vi "Write Graph Properties.vi"(0 "Config File":path, 7 "WFGraph Refnum":refnum<vi>, 9 "Section":string, 11 "error in (no error)":errorcluster) -> (15 "error out":errorcluster)   [LabVIEW 2020]
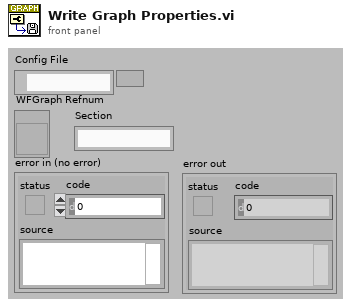
[diagram p1: front panel]
types:
  T1 = typedef "Graph Properties.ctl" = cluster{"X-axis":T2, "Y-axis":T2, "Plot Properties":T3[]}
  T2 = typedef "Axis Properties.ctl" = cluster{"Min":dbl, "Max":dbl, "Fit":u8}
  T3 = typedef "Plot Properties.ctl" = cluster{"Line Style":u8, "Line Width":u8, "Plot Color":u32, "Point Style":u8, "Point color":u32, "Interp":u8}
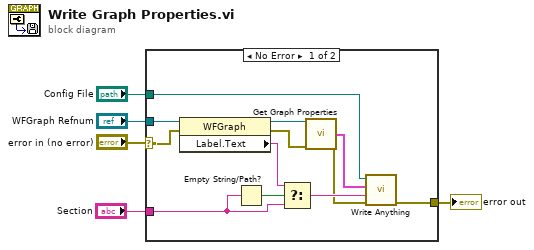
[diagram p0: block diagram]
diagram:
  n1 = case shown="No Error" "error in (no error)" {
    selector: "error in (no error)" -> [w16 w18]
    tunnel: "WFGraph Refnum" -> [w17 _]
    tunnel: "Config File" -> [w15 _]
    tunnel: [w14 w18] -> w2
    tunnel: "Section" -> [w11 _]
    frame No Error {
      n2 = property class="WFGraph"(reference=w17, error in=w16) -> (reference out=w9:refnum<vi>, error out=w8:errorcluster, "Label.Text"=w12:string)
      n3 = Empty String/Path?(string/path=w11) -> (empty?=w13:bool)
      n4 = Select(t=w12, s=w13, f=w11) -> (s? t:f=w10:string)
      n5 = call "Get Graph Properties.vi"("WFGraph Refnum"=w9, "error in (no error)"=w8) -> ("Graph Properties"=w6:T1, "error out"=w7:errorcluster)  [unwired: 11 in, 1 out]
      n6 = call "Write Anything.vi"("Error In"=w7, "Section Name (Name of \"Anything\")"=w10, "Anything"=w6, "Path (dialog)"=w15) -> ("Error Out"=w14:errorcluster)  [unwired: 6 in, 1 out]
    }
    frame Error {
    }
  }
  "error out" <- w2
